vi "Send Show Pane Settings UI.vi"(7 "Message Priority (Normal)":T1=enum."Normal", 8 "error in (no error)":errorcluster, 10 "Pane":refnum<class "Pane.lvclass">, 11 "Message Enqueuer":refnum<class "Message Enqueuer.lvclass">) -> (0 "error out":errorcluster, 3 "Message Enqueuer out":refnum<class "Message Enqueuer.lvclass">)   [LabVIEW 2018, in "Pane Settings UI.lvlib" / "Show Pane Settings UI Msg.lvclass"]
doc: "This VI sends the message to an actor."
uses:
  <resource>/dialog/QuickDrop/plugins/PaneRelief/Classes/Pane Settings UI/Pane Settings UI Messages/Show Pane Settings UI Msg/Show Pane Settings UI Msg.lvclass
  <vilib>/ActorFramework/Message Enqueuer/Message Enqueuer.lvclass
  <vilib>/ActorFramework/Message Enqueuer/Message Priority.ctl
  <resource>/dialog/QuickDrop/plugins/PaneRelief/Classes/Pane/Pane.lvclass
  C:/Program Files (x86)/National Instruments/LabVIEW 2018/vi.lib/ActorFramework/Message/Message.lvclass
  <resource>/dialog/QuickDrop/plugins/PaneRelief/Classes/Pane Settings UI/Pane Settings UI Messages/Show Pane Settings UI Msg/Show Pane Settings UI Msg.lvclass/Show Pane Settings UI Msg.ctl
  <vilib>/ActorFramework/Message Enqueuer/Message Enqueuer.lvclass/Message Enqueuer.ctl
  <vilib>/ActorFramework/Message Priority Queue/Priority Enqueue.vi
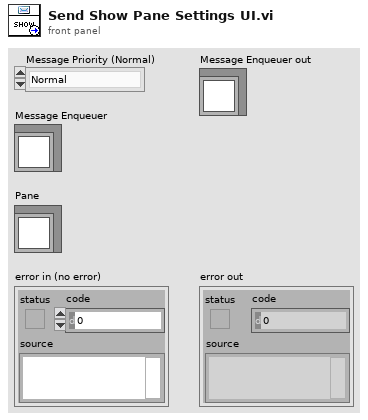
[diagram p1: front panel]
types:
  T1 = typedef "Actor Framework.lvlib/Message Enqueuer.lvclass/Message Priority.ctl" = enum16{"Low", "Normal", "High"}
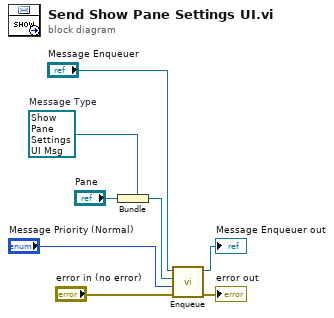
[diagram p0: block diagram]
diagram:
  w5 = refnum<class "Show Pane Settings UI Msg.lvclass"> refnum  # Message Type
  n1 = Bundle(cluster=w5, "Pane") -> (w4:refnum<class "Show Pane Settings UI Msg.lvclass">)
  n2 = call <vilib>:"Enqueue.vi"("error in (no error)"="error in (no error)", "Message Priority (Normal)"="Message Priority (Normal)", "Message"=w4, "Message Enqueuer in"="Message Enqueuer") -> ("error out"=→"error out":errorcluster, "Message Enqueuer out"=→"Message Enqueuer out":refnum<class "Message Enqueuer.lvclass">)  [unwired: 6 in]
